vi "uTTA_GetSystemTime.vi"(4 "error in":errorcluster, 7 "VISA Refnum in":refnum<visa-resource-name>) -> (0 "error out":errorcluster, 1 "Timestamp":timestamp, 2 "Received":string, 3 "VISA Refnum out":refnum<visa-resource-name>)   [LabVIEW 2021]
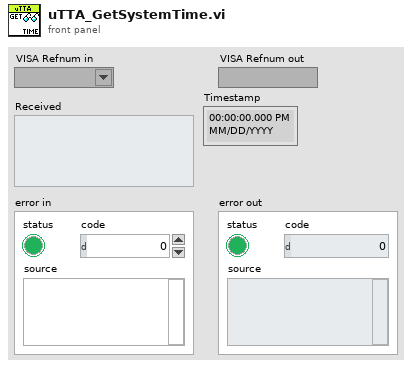
[diagram p1: front panel]
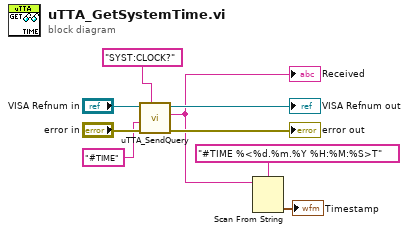
[diagram p0: block diagram]
diagram:
  n1 = call "uTTA_SendQuery.vi"("Send String"="SYST:CLOCK?" ("format string"), "error in (no error)"="error in", "Response Qualifier(\"\")"="#TIME" ("Response Qualifier(\"\")"), "VISA Refnum in"="VISA Refnum in") -> ("error out"=→"error out":errorcluster, "Received"=w3:string, "VISA Refnum out"=→"VISA Refnum out":refnum<visa-resource-name>)  [unwired: 5 in]
  "Received" <- w3
  n2 = Scan From String(format string="#TIME %<%d.%m.%Y %H:%M:%S>T", input string=w3) -> (output 1=→"Timestamp":timestamp)  [unwired: 3 in, 3 out]
